vi "Update LHW Data.vi"(8 "Error In":errorcluster, 10 "LHW-DataCollection":refnum<class "LHW-DataCollection.lvclass">, 11 "LHW-GUI-Actor in":refnum<class "LHW-GUI-Actor.lvclass">) -> (0 "Error Out":errorcluster, 3 "LHW-GUI-Actor out":refnum<class "LHW-GUI-Actor.lvclass">)   [LabVIEW 2014, in "LHW-GUI.lvlib" / "LHW-GUI-Actor.lvclass"]
doc: "Update LHW Data on GUI."
uses:
  LHW-GUI-Actor.lvclass
  Classes/LHW-Data/LHW-DataCollection/LHW-DataCollection.lvclass
  Classes/LHW-Data/LHW-DataCollection/LHW-DataCollection.lvclass/LHW-DataCollection.ctl
  LHW-GUI-Actor.lvclass/LHW-GUI-Actor.ctl
  LHW-Analysis-Actor Messages/Analyze Msg/Analyze Msg.lvclass/Analyze Msg.ctl
  <vilib>/ActorFramework/Message Enqueuer/Message Enqueuer.lvclass/Message Enqueuer.ctl
  LHW-Storage-Actor Messages/Store Data Msg/Store Data Msg.lvclass/Store Data Msg.ctl
  <vilib>/ActorFramework/Message Enqueuer/Enqueue.vi
  <vilib>/ActorFramework/Message Priority Queue/Priority Enqueue.vi
  Classes/LHW-Data/LHW-Data/LHW-Data.lvclass
  <vilib>/ActorFramework/Message Enqueuer/Message Enqueuer.lvclass
  LHW-Analysis-Actor Messages/Analyze Msg/Analyze Msg.lvclass
  LHW-Storage-Actor Messages/Store Data Msg/Store Data Msg.lvclass
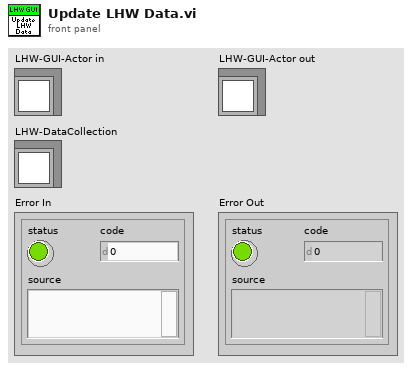
[diagram p1: front panel]
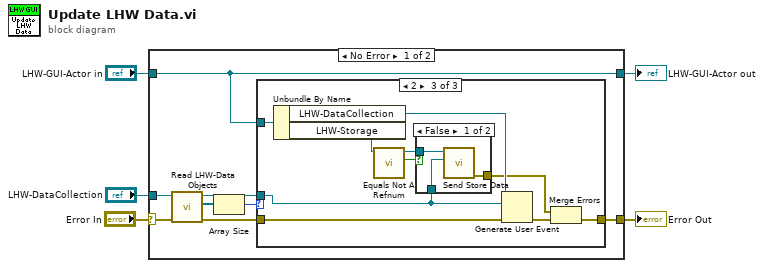
[diagram p0: block diagram]
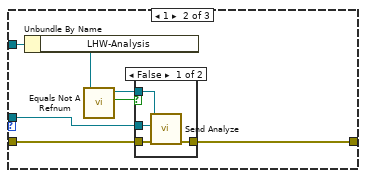
[diagram p3: hidden frame]
diagram:
  n1 = case shown="No Error" "Error In" {
    selector: "Error In" -> [w9 w39]
    tunnel: [w12 w39] -> w4
    tunnel: [w13 w38] -> w2
    tunnel: "LHW-GUI-Actor in" -> [w13 w38]
    tunnel: "LHW-DataCollection" -> [w11 _]
    frame No Error {
      n2 = call "Read LHW-Data Objects.vi"("error in (no error)"=w9, "LHW-DataCollection in"=w11) -> ("error out"=w8:errorcluster, "LHW-Data Objects"=w7:refnum<class "LHW-Data.lvclass">[], "LHW-DataCollection out"=w10:refnum<class "LHW-DataCollection.lvclass">)  [unwired: 7 in]
      n3 = Array Size(array=w7) -> (size(s)=w6:i32)
      n4 = case shown="2" w6 {
        tunnel: w13 -> [_ w20 w34]
        tunnel: [w14 w15 w27] -> w12
        tunnel: w10 -> [_ w19 w29]
        tunnel: w8 -> [w14 w18 w31]
        frame Default {
        }
        frame 1 {
          n5 = Unbundle By Name(w20) -> ("LHW-Analysis"=w17:refnum<class "Message Enqueuer.lvclass">)
          n6 = call <vilib>:"Equals Not A Refnum.vi"("Message Enqueuer"=w17) -> ("Not a refnum?"=w16:bool)  [unwired: 10 in]
          n7 = case shown="False" w16 {
            tunnel: w19 -> [w24 _]
            tunnel: w18 -> [w23 w25]
            tunnel: w17 -> [w22 _]
            tunnel: [w21 w25] -> w15
            frame False {
              n8 = call "Send Analyze.vi"("error in (no error)"=w23, "LHW-DataCollection"=w24, "Message Enqueuer"=w22) -> ("error out"=w21:errorcluster)  [unwired: 7 in, 1 out]
            }
            frame True {
            }
          }
        }
        frame 2 {
          n9 = Unbundle By Name(w34) -> ("LHW-DataCollection"=w33:refnum<user-event>, "LHW-Storage"=w30:refnum<class "Message Enqueuer.lvclass">)
          n10 = call <vilib>:"Equals Not A Refnum.vi"("Message Enqueuer"=w30) -> ("Not a refnum?"=w28:bool)  [unwired: 10 in]
          n11 = case shown="False" w28 {
            tunnel: w30 -> [w37 _]
            tunnel: w29 -> [w36 _]
            tunnel: [w35 _] -> w26
            frame False {
              n12 = call "Send Store Data.vi"("LHW-DataCollection"=w36, "Message Enqueuer"=w37) -> ("error out"=w35:errorcluster)  [unwired: 8 in, 1 out]
            }
            frame True {
            }
          }
          n13 = Generate User Event(user event=w33, event data cluster=w29, error in=w31) -> (error out=w32:errorcluster)  [unwired: 1 in, 1 out]
          n14 = Merge Errors(w26, w32) -> (w27:errorcluster)
        }
      }
    }
    frame Error {
    }
  }
  "Error Out" <- w4
  "LHW-GUI-Actor out" <- w2
